vi "J1939 Editor.vi"() -> ()   [LabVIEW 2013]
doc: "This is the main VI for the configuration editor."
uses:
  Controls/StateCluster.ctl
  <vilib>/NI/Configuration Framework/Repository/NISE_CEF_Repository.lvclass
  <vilib>/NI/Configuration Framework/Node/NodeRef.ctl
  <vilib>/NI/Configuration Framework/Node/NISE_CEF_Node.lvclass
  <vilib>/NI/Configuration Framework/Node/UserEventRef.ctl
  <vilib>/NI/Configuration Framework/Controls/EventCluster.ctl
  Controls/AddMessage.ctl
  Controls/MoveMessage.ctl
  Classes/can port/can port.lvclass
  Classes/database file/database file.lvclass
  <vilib>/NI/AMC/Read Termination Message.vi
  <vilib>/NI/AMC/Create Single Message.vi
  <vilib>/NI/AMC/Update Message Routing Info.vi
  <vilib>/NI/AMC/Send Message.vi
  <vilib>/NI/AMC/Globals.vi
  <vilib>/NI/AMC/AMC.lvlib
  <vilib>/NI/Configuration Framework/NISE_CEF_TreeControl.lvlib
panel:
  in  "View":string(tree)
  in  "Exit":bool
  # "J1939 Device Configurator"
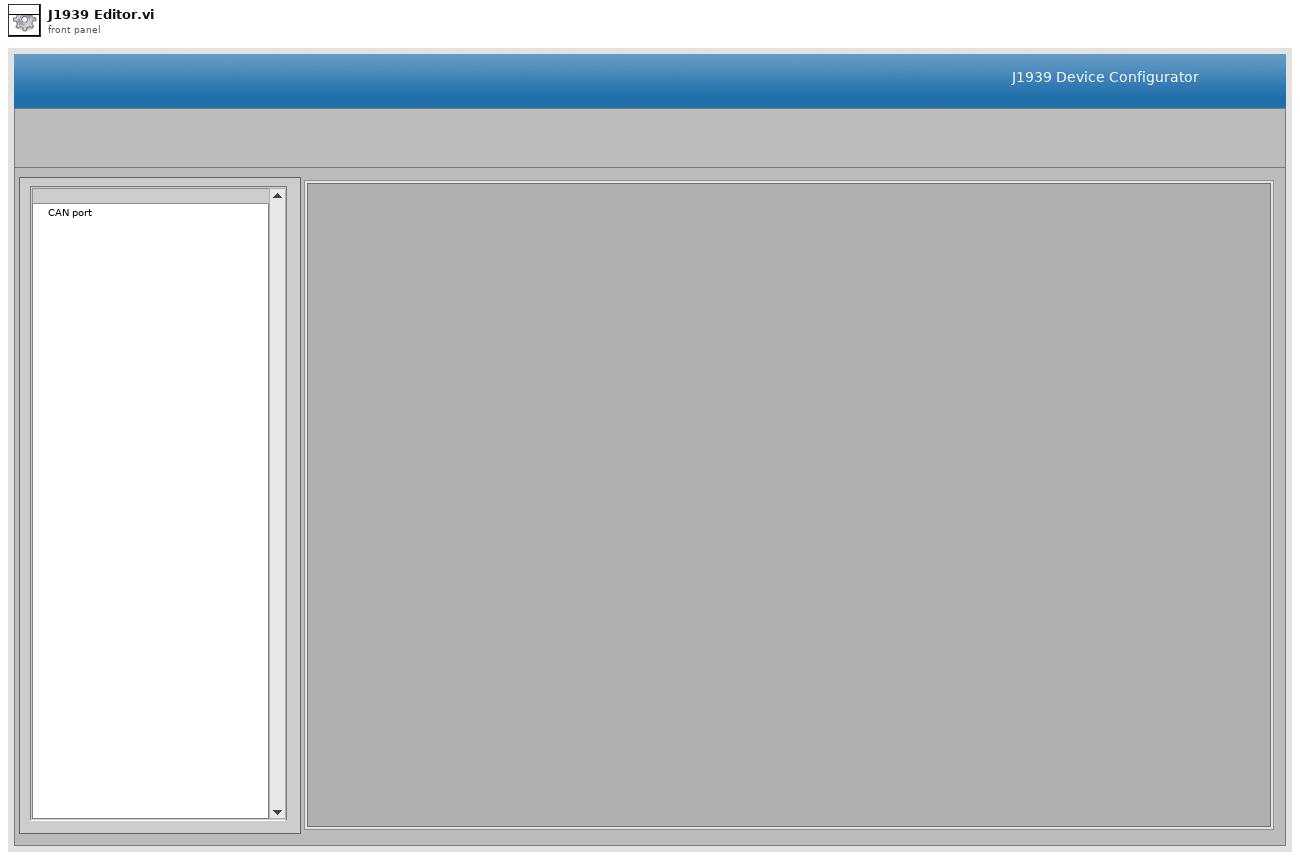
[diagram p1: front panel]
types:
  T1 = typedef "StateCluster.ctl" = cluster{"repository":refnum<class "NISE_CEF_Repository.lvclass">, "root":T2, "unsaved changes":bool, "current path":path, "user event ref":T3, "glyph path":path, "classes path":path}
  T2 = typedef "NISE_CEF_Node.lvclass/NodeRef.ctl" = refnum<data-value>
  T3 = typedef "NISE_CEF_Node.lvclass/UserEventRef.ctl" = refnum<user-event>
  T4 = typedef "AMC.lvlib/Message Queue.ctl" = refnum<queue>
  T5 = typedef "AddMessage.ctl" = cluster{"node type":string, "to add to":string}
  T6 = typedef "MoveMessage.ctl" = cluster{"node ref":T2, "new parent":T2}
  T7 = typedef "NISE_CEF_TreeControl.lvlib/EventCluster.ctl" = cluster{"command":string, "data":string}
  T8 = typedef "FilePaths.ctl" = cluster{"glyphs":path, "classes":path}
  T9 = typedef "NISE_CEF_Node.lvclass/Summary.ctl" = cluster{"ID":string, "parent ID":string, "node type":string, "text":string, "additional text":string, "glyph":string, "depth":i32, "glyph overlay":string}
  T10 = typedef "LVPoint32TypeDef.ctl" = cluster{"Horizontal":i32, "Vertical":i32}
  T11 = cluster{"data name":string, "drag data":variant}[]
  T12 = typedef "NISE_CEF_Node.lvclass/NodeMenuOptions.ctl" = cluster{"removable":bool, "movable":bool, "duplicate":bool}
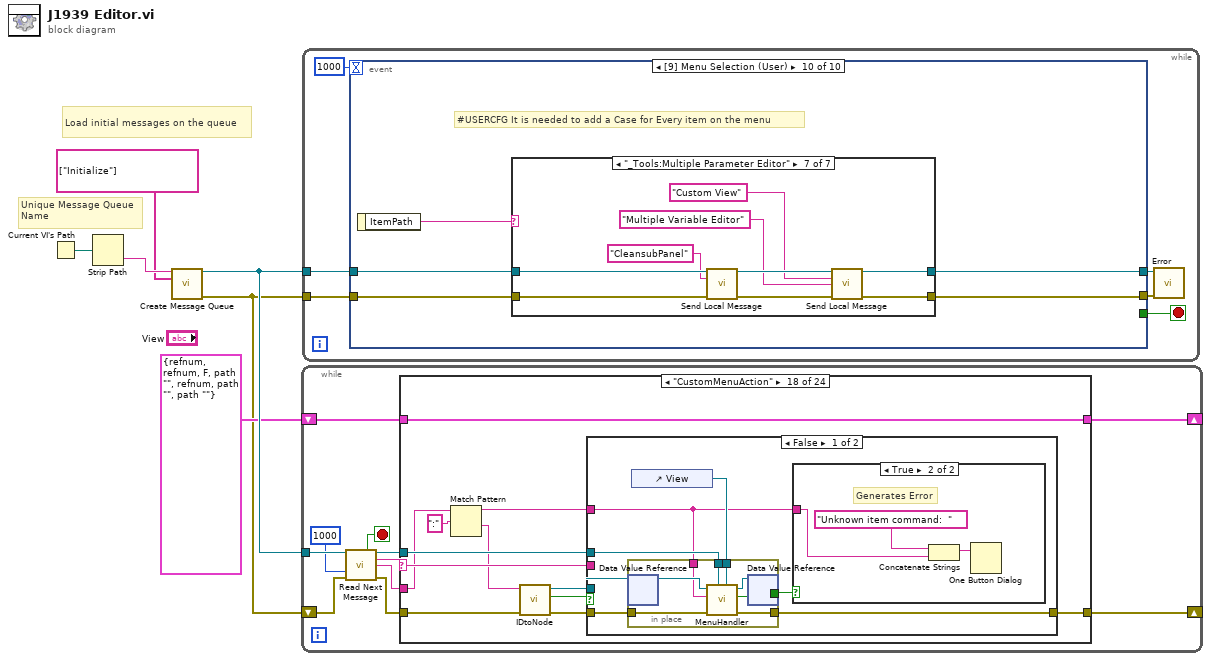
[diagram p0: block diagram]
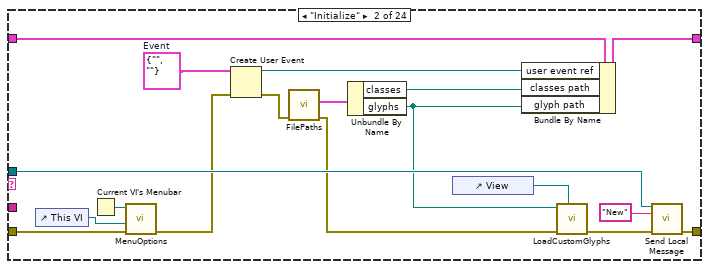
[diagram p3: hidden frame]
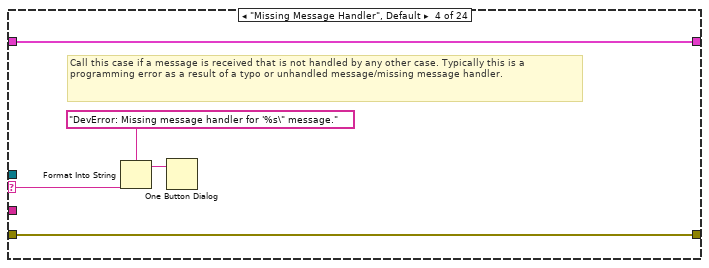
[diagram p5: hidden frame]
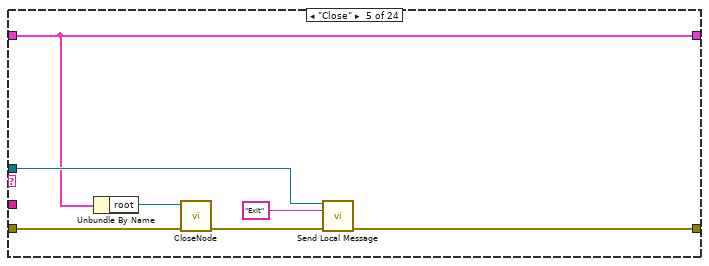
[diagram p6: hidden frame]
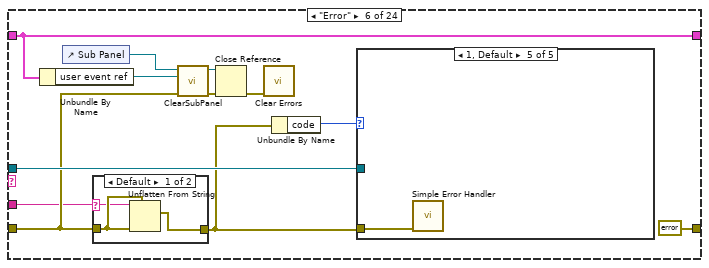
[diagram p7: hidden frame]
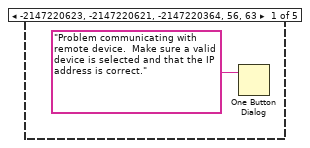
[diagram p9: hidden frame]
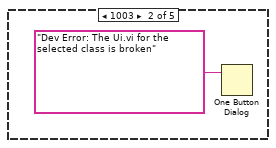
[diagram p10: hidden frame]
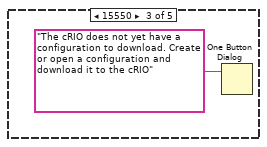
[diagram p11: hidden frame]
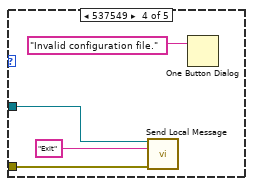
[diagram p12: hidden frame]
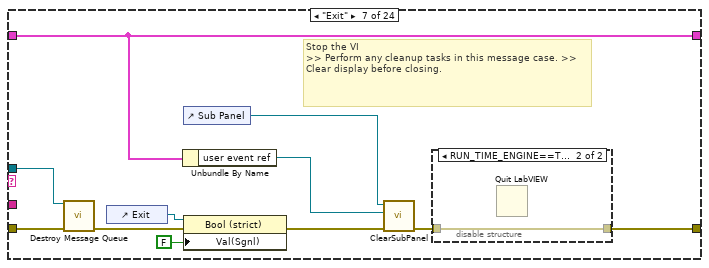
[diagram p13: hidden frame]
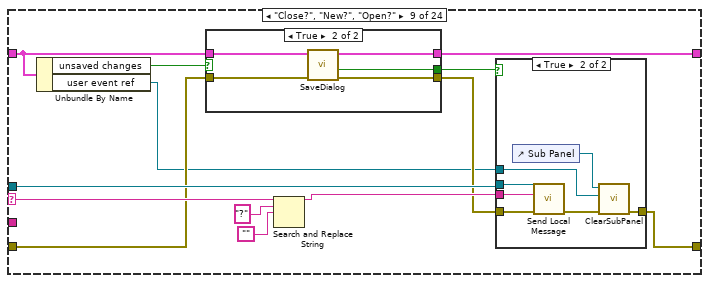
[diagram p16: hidden frame]
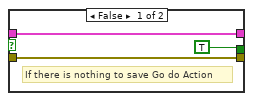
[diagram p17: hidden frame]
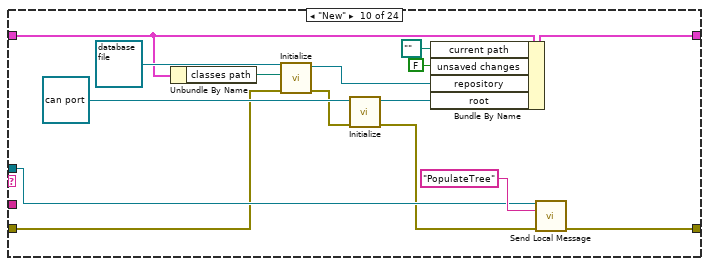
[diagram p19: hidden frame]
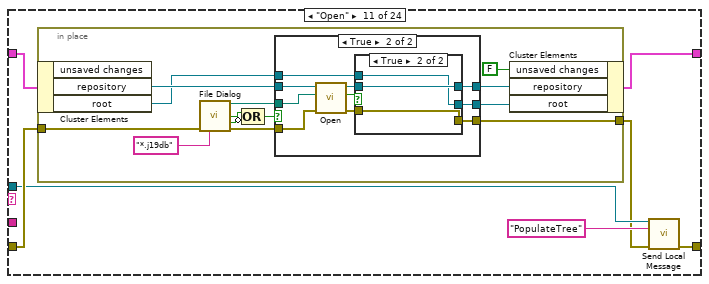
[diagram p20: hidden frame]
diagram:
  # "Unique Message Queue Name"
  # "Load initial messages on the queue"
  n1 = Current VI's Path() -> (path=w5:path)
  n2 = Strip Path(path=w5) -> (name=w6:string)  [unwired: 1 out]
  n3 = call <vilib>:"Create Message Queue.vi"("message queue name"=w6, "initial message names"=string[] ["Initialize"]) -> ("message queue out"=w3:T4, "error out"=w1:errorcluster)  [unwired: 12 in]
  n4 = while "Message Processor" {
    shift-right: [w13] -> _
    shift-left: w1 -> [w12]
    tunnel: w3 -> [w11]
    shift-right: [w9] -> _
    shift-left: T1 {"repository"=refnum, "root"=refnum, "unsaved changes"=FALSE, "current path"=path "", "user event ref"=refnum, "glyph path"=path "", "classes path"=path ""} -> [w8]
    stop <- w17 stop-if-true
    n5 = call <vilib>:"Read Next Message.vi"("message queue in"=w11, "timeout (1 ms)"=1000, "error in"=w12) -> ("exit process?"=w17:bool, "message queue out"=w7:T4, "message name"=w16:string, "message value"=w15:string, "error out"=w14:errorcluster)  [unwired: 5 in, 3 out]
    n6 = case shown="\"CustomMenuAction\"" w16 {
      selector: w16 -> [_ _ _ w41 _ _ _ _ w99 _ _ _ _ _ _ _ _ w279 _ _ _ _ _ _]
      tunnel: w15 -> [_ _ _ _ _ w52 _ _ _ _ _ _ _ w212 _ w249 w260 w277 w308 w329 _ _ w365 w385]
      tunnel: w14 -> [w19 w37 w39 w44 w46 w55 w86 w90 w92 w121 w139 w178 w204 w219 w232 w238 w259 w282 w310 w328 w345 w355 w364 w383]
      tunnel: [w19 w31 w39 w44 w50 errorcluster {"status"=FALSE, "code"=0, "source"=""} ("error out") w78 w90 w103 w133 w135 w182 w206 w216 w232 w241 w263 w285 w314 w325 w339 w350 w361 w378] -> w13
      tunnel: [w18 w26 w38 w40 w48 w60 w77 w89 w94 w131 w140 w185 w205 w213 w231 w235 w264 w286 w312 w330 w349 w354 w359 w386] -> w9
      tunnel: w8 -> [w18 w27 w38 w40 w48 w60 w77 w89 w95 w125 w141 w180 w203 w214 w231 w236 w264 w286 w313 w330 w349 w354 w359 w386]
      tunnel: w7 -> [_ w30 _ _ w49 w63 w85 _ w102 w132 w137 w181 _ w215 _ _ _ w280 _ _ _ _ w360 w377]
      frame "------------Generic Operations------------" {
        # "Dummy case to add a seperation in the Case Structure menu"
      }
      frame "Initialize" {
        w21 = T7 {"command"="", "data"=""}  # Event
        n7 = control-ref of="This VI"() -> (w36:refnum<vi>)
        n8 = Current VI's Menubar() -> (w35:refnum<k9>)
        n9 = call "MenuOptions.vi"("error in"=w37, "VI ref"=w36, "menu ref in"=w35) -> ("error out"=w25:errorcluster)  [unwired: 7 in, 1 out]
        n10 = Create User Event(user event datatype=w21, error in=w25) -> (user event=w20:refnum<user-event>, error out=w24:errorcluster)
        n11 = call "FilePaths.vi"("error in"=w24) -> ("error out"=w29:errorcluster, "paths"=w28:T8)  [unwired: 9 in]
        n12 = Unbundle By Name(w28) -> ("classes"=w23:path, "glyphs"=w22:path)
        n13 = control-ref of="View"() -> (w34:refnum<vi>)
        n14 = Bundle By Name(cluster=w27, "user event ref"=w20, "classes path"=w23, "glyph path"=w22) -> (w26:T1)
        n15 = call <vilib>:"LoadCustomGlyphs.vi"("tree ref"=w34, "error in"=w29, "glyph directory"=w22) -> ("error out"=w32:errorcluster)  [unwired: 8 in]
        n16 = call <vilib>:"Send Local Message.vi"("message queue in"=w30, "message name"="New" ("Message Name"), "error in"=w32) -> ("error out"=w31:errorcluster)  [unwired: 10 in, 2 out]
      }
      frame "", "Idle" {
      }
      frame "Missing Message Handler", Default {
        # "Call this case if a message is received that is not handled by any other case. Typically this is a programming error as a result of a typo or unhandled message/missing message handler."
        n17 = Format Into String(format string="DevError: Missing message handler for '%s\" message." ("message"), w41) -> (resulting string=w43:string)  [unwired: 2 in, 1 out]
        n18 = One Button Dialog(message=w43) -> ()  [unwired: 2 out]
      }
      frame "Close" {
        n19 = Unbundle By Name(w48) -> ("root"=w47:T2)
        n20 = call <vilib>:"CloseNode.vi"("error in"=w46, "node ref"=w47) -> ("error out"=w45:errorcluster)  [unwired: 9 in]
        n21 = call <vilib>:"Send Local Message.vi"("message queue in"=w49, "message name"="Exit", "error in"=w45) -> ("error out"=w50:errorcluster)  [unwired: 10 in, 2 out]
      }
      frame "Error" {
        n22 = Unbundle By Name(w60) -> ("user event ref"=w58:T3)
        n23 = control-ref of="Sub Panel"() -> (w59:refnum<vi>)
        n24 = case shown="Default" w52 {
          selector: w52 -> [w65 _]
          tunnel: w55 -> [w66 w67]
          tunnel: [w64 w67] -> w54
          frame Default {
            n25 = Unflatten From String(type=w66, binary string=w65, error in (no error)=w66) -> (value=w64:errorcluster)  [unwired: 2 in, 2 out]
          }
          frame "" {
          }
        }
        n26 = call <vilib>:"ClearSubPanel.vi"("error in"=w55, "user event ref"=w58, "sub panel ref in"=w59) -> ("error out"=w57:errorcluster, "sub panel ref out"=w56:refnum<vi>)  [unwired: 7 in]
        n27 = Close Reference(reference=w56, error in (no error)=w57) -> (error out=w53:errorcluster)
        n28 = call <vilib>:"Clear Errors.vi"("error in (no error)"=w53) -> ()  [unwired: 6 in, 1 out]
        n29 = Unbundle By Name(w54) -> ("code"=w61:i32)
        n30 = case shown="1, Default" w61 {
          tunnel: w63 -> [_ _ _ w73 _]
          tunnel: w54 -> [_ _ _ w72 w75]
          frame -2147220623, -2147220621, -2147220364, 56, 63 {
            n31 = One Button Dialog(message="Problem communicating with remote device.  Make sure a valid device is selected and that the IP address is correct.") -> ()  [unwired: 1 in, 1 out]
          }
          frame 1003 {
            n32 = One Button Dialog(message="Dev Error: The Ui.vi for the selected class is broken") -> ()  [unwired: 1 in, 1 out]
          }
          frame 15550 {
            n33 = One Button Dialog(message="The cRIO does not yet have a configuration to download. Create or open a configuration and download it to the cRIO") -> ()  [unwired: 1 in, 1 out]
          }
          frame 537549 {
            n34 = call <vilib>:"Send Local Message.vi"("message queue in"=w73, "message name"="Exit", "error in"=w72) -> ()  [unwired: 10 in, 3 out]
            n35 = One Button Dialog(message="Invalid configuration file.") -> ()  [unwired: 1 in, 1 out]
          }
          frame 1, Default {
            n36 = call <vilib>:"Simple Error Handler.vi"("error in (no error)"=w75) -> ()  [unwired: 1 in, 8 out]
          }
        }
      }
      frame "Exit" {
        # "Stop the VI                                                                             >> Perform any cleanup tasks in this message case. >> Clear display before closing."
        n37 = call <vilib>:"Destroy Message Queue.vi"("message queue in"=w85, "error in"=w86) -> ("error out"=w82:errorcluster)  [unwired: 11 in, 2 out]
        n38 = control-ref of="Exit"() -> (w84:refnum<vi>)
        n39 = Unbundle By Name(w77) -> ("user event ref"=w76:T3)
        n40 = control-ref of="Sub Panel"() -> (w81:refnum<vi>)
        n41 = property class="Bool (strict)"(reference=w84, error in=w82, "Val(Sgnl)"=FALSE ("Exit")) -> (error out=w80:errorcluster)  [unwired: 1 out]
        n42 = call <vilib>:"ClearSubPanel.vi"("error in"=w80, "user event ref"=w76, "sub panel ref in"=w81) -> ("error out"=w79:errorcluster)  [unwired: 7 in, 1 out]
        n43 = disable-structure shown="RUN_TIME_ENGINE==True" {
          disable-tunnel: [w87 w88] -> w78
          disable-tunnel: w79 -> [w87 w88]
          frame condition #0 (active) {
          }
          frame condition #1 {
            n44 = Quit LabVIEW() -> ()  [unwired: 1 in]
          }
        }
      }
      frame "------------Menu Operations--------------" {
        # "Dummy case to add a seperation in the Case Structure menu"
      }
      frame "Close?", "New?", "Open?" {
        n45 = Unbundle By Name(w95) -> ("unsaved changes"=w97:bool, "user event ref"=w91:T3)
        n46 = case shown="True" w97 {
          tunnel: [TRUE ("SaveFlag") w111] -> w96
          tunnel: w95 -> [w105 w110]
          tunnel: [w105 w109] -> w94
          tunnel: w92 -> [w104 w108]
          tunnel: [w104 w107] -> w93
          frame False {
            # "If there is nothing to save Go do Action"
          }
          frame True {
            n47 = call "SaveDialog.vi"("error in"=w108, "state in"=w110) -> ("error out"=w107:errorcluster, "new"=w111:bool, "state out"=w109:T1)  [unwired: 7 in]
          }
        }
        n48 = Search and Replace String(input string=w99, search string="?", replace string="") -> (result string=w98:string)  [unwired: 5 in, 3 out]
        n49 = case shown="True" w96 {
          tunnel: w93 -> [w112 w119]
          tunnel: [w112 w115] -> w103
          tunnel: w102 -> [_ w118]
          tunnel: w98 -> [_ w117]
          tunnel: w91 -> [_ w114]
          frame False {
          }
          frame True {
            n50 = control-ref of="Sub Panel"() -> (w113:refnum<vi>)
            n51 = call <vilib>:"Send Local Message.vi"("message queue in"=w118, "message name"=w117, "error in"=w119) -> ("error out"=w116:errorcluster)  [unwired: 10 in, 2 out]
            n52 = call <vilib>:"ClearSubPanel.vi"("error in"=w116, "user event ref"=w114, "sub panel ref in"=w113) -> ("error out"=w115:errorcluster)  [unwired: 7 in, 1 out]
          }
        }
      }
      frame "New" {
        n53 = Unbundle By Name(w125) -> ("classes path"=w124:path)
        n54 = call-dynamic "Initialize.vi"("error in"=w121, "path"=w124, "repository in"=refnum<class "database file.lvclass"> refnum ("cRIORepo.lvclass")) -> ("error out"=w123:errorcluster, "repository out"=w126:refnum<class "database file.lvclass">)  [unwired: 7 in]
        n55 = call-dynamic "Initialize.vi"("error in"=w123, "cRIO in"=refnum<class "can port.lvclass"> refnum ("cRIO.lvclass")) -> ("error out"=w122:errorcluster, "data value reference"=w128:T2)  [unwired: 7 in, 1 out]
        n56 = Bundle By Name(cluster=w125, "current path"=path "", "unsaved changes"=FALSE ("SaveFlag"), "repository"=w126, "root"=w128) -> (w131:T1)
        n57 = call <vilib>:"Send Local Message.vi"("message queue in"=w132, "message name"="PopulateTree", "error in"=w122) -> ("error out"=w133:errorcluster)  [unwired: 10 in, 2 out]
      }
      frame "Open" {
        n58 = in-place {
          in-place-border: w139 -> [w147]
          in-place-border: [w151] -> w136
          n59 = in-place-cluster #1(w141) -> ("repository"=w154:refnum<class "NISE_CEF_Repository.lvclass">, "root"=w145:T2)  [unwired: 1 out]
          n60 = call "File Dialog"("error in"=w147, "pattern (all files)"="*.j19db") -> ("selected path"=w148:path, "exists"=w144:bool, "cancelled"=w143:bool, "error out"=w146:errorcluster)  [unwired: 10 in]
          n61 = Compound Arithmetic op=OR(w144, invert w143) -> (w142:bool)
          n62 = case shown="True" w142 {
            tunnel: w154 -> [w155 w167]
            tunnel: [w155 w165] -> w152
            tunnel: [w156 w163] -> w151
            tunnel: [w157 w162] -> w150
            tunnel: w148 -> [_ w160]
            tunnel: w146 -> [w156 w159]
            tunnel: w145 -> [w157 w158]
            frame False {
            }
            frame True {
              n63 = call-dynamic "Open.vi"("error in"=w159, "file path"=w160, "repository in"=w167) -> ("error out"=w164:errorcluster, "invalid?"=w161:bool, "repository out"=w166:refnum<class "NISE_CEF_Repository.lvclass">)  [unwired: 6 in]
              n64 = case shown="True" w161 {
                tunnel: w166 -> [w172 w175]
                tunnel: [w171 w175] -> w165
                tunnel: w164 -> [w170 w174]
                tunnel: [w169 w174] -> w163
                tunnel: [w168 w173] -> w162
                tunnel: w158 -> [_ w173]
                frame False {
                  n65 = call-dynamic "WriteTree.vi"("error in"=w170, "repository in"=w172) -> ("error out"=w169:errorcluster, "root"=w168:T2, "repository out"=w171:refnum<class "NISE_CEF_Repository.lvclass">)  [unwired: 7 in]
                }
                frame True {
                }
              }
            }
          }
          n66 = in-place-cluster #1("unsaved changes"=FALSE ("SaveFlag"), "repository"=w152, "root"=w150) -> (w140:T1)
        }
        n67 = call <vilib>:"Send Local Message.vi"("message queue in"=w137, "message name"="PopulateTree", "error in"=w136) -> ("error out"=w135:errorcluster)  [unwired: 10 in, 2 out]
      }
      frame "Save" {
        n68 = in-place {
          in-place-border: w178 -> [w189]
          in-place-border: [w188] -> w177
          in-place-border: [w186] -> w176
          n69 = in-place-cluster #2(w180) -> ("current path"=w187:path, "root"=w190:T2, "repository"=w192:refnum<class "NISE_CEF_Repository.lvclass">)
          n70 = Empty String/Path?(string/path=w187) -> (empty?=w186:bool)
          n71 = call-dynamic "ReadTree.vi"("error in"=w189, "root"=w190, "repository in"=w192) -> ("error out"=w188:errorcluster, "repository out"=w191:refnum<class "NISE_CEF_Repository.lvclass">)  [unwired: 7 in]
          n72 = in-place-cluster #2("current path"=w187, "root"=w190, "repository"=w191) -> (w179:T1)
        }
        n73 = case shown="True" w176 {
          tunnel: w179 -> [w196 w198]
          tunnel: [w195 w197] -> w185
          tunnel: [w194 w199] -> w183
          tunnel: w177 -> [w193 w200]
          frame False {
            n74 = call "Save.vi"("error in"=w193, "state in"=w196) -> ("error out"=w194:errorcluster, "state out"=w195:T1)  [unwired: 8 in]
          }
          frame True {
            # "Empty path use Dialog"
            n75 = call "SaveAs.vi"("error in"=w200, "state in"=w198) -> ("error out"=w199:errorcluster, "state out"=w197:T1)  [unwired: 7 in, 1 out]
          }
        }
        n76 = call <vilib>:"Send Local Message.vi"("message queue in"=w181, "message name"="PopulateTree", "error in"=w183) -> ("error out"=w182:errorcluster)  [unwired: 10 in, 2 out]
      }
      frame "SaveAs" {
        n77 = in-place {
          in-place-border: w204 -> [w208]
          in-place-border: [w207] -> w202
          n78 = in-place-cluster #3(w203) -> ("root"=w209:T2, "repository"=w211:refnum<class "NISE_CEF_Repository.lvclass">)
          n79 = call-dynamic "ReadTree.vi"("error in"=w208, "root"=w209, "repository in"=w211) -> ("error out"=w207:errorcluster, "repository out"=w210:refnum<class "NISE_CEF_Repository.lvclass">)  [unwired: 7 in]
          n80 = in-place-cluster #3("root"=w209, "repository"=w210) -> (w201:T1)
        }
        n81 = call "SaveAs.vi"("error in"=w202, "state in"=w201) -> ("error out"=w206:errorcluster, "state out"=w205:T1)  [unwired: 7 in, 1 out]
      }
      frame "Custom View" {
        n82 = in-place {
          in-place-border: w219 -> [w230]
          in-place-border: [w229] -> w217
          in-place-border: w212 -> [w220]
          n83 = in-place-cluster #4(w214) -> ("repository"=w224:refnum<class "NISE_CEF_Repository.lvclass">, "root"=w223:T2)
          n84 = call-dynamic "ReadTree.vi"("error in"=w230, "root"=w223, "repository in"=w224) -> ("error out"=w227:errorcluster, "repository out"=w226:refnum<class "NISE_CEF_Repository.lvclass">)  [unwired: 7 in]
          n85 = call-dynamic "CustomView.vi"("error in"=w227, "view name"=w220, "repository in"=w226) -> ("error out"=w228:errorcluster, "repository out"=w225:refnum<class "NISE_CEF_Repository.lvclass">)  [unwired: 7 in]
          n86 = call-dynamic "WriteTree.vi"("error in"=w228, "repository in"=w225) -> ("error out"=w229:errorcluster, "root"=w221:T2, "repository out"=w222:refnum<class "NISE_CEF_Repository.lvclass">)  [unwired: 7 in]
          n87 = in-place-cluster #4("repository"=w222, "root"=w221) -> (w213:T1)
        }
        n88 = call <vilib>:"Send Local Message.vi"("message queue in"=w215, "message name"="PopulateTree", "error in"=w217) -> ("error out"=w216:errorcluster)  [unwired: 10 in, 2 out]
      }
      frame "-------TreeControl Operations-----------" {
        # "Dummy case to add a seperation in the Case Structure menu"
      }
      frame "AddNode" {
        n89 = Unflatten From String(type=T5 {"node type"="", "to add to"=""} ("input cluster"), binary string=w249) -> (value=w247:T5)  [unwired: 3 in, 2 out]
        n90 = Unbundle By Name(w247) -> ("to add to"=w244:string, "node type"=w234:string)
        n91 = in-place {
          in-place-border: w238 -> [w255]
          in-place-border: [w254] -> w237
          in-place-border: w234 -> [w253]
          in-place-border: [w252] -> w233
          n92 = in-place-cluster #5(w236) -> ("repository"=w257:refnum<class "NISE_CEF_Repository.lvclass">)
          n93 = call-dynamic "GetClassPath.vi"("error in"=w255, "class name"=w253, "Repository in"=w257) -> ("error out"=w254:errorcluster, "class path"=w252:path, "Repository out"=w256:refnum<class "NISE_CEF_Repository.lvclass">)  [unwired: 6 in]
          n94 = in-place-cluster #5("repository"=w256) -> (w235:T1)
        }
        n95 = control-ref of="View"() -> (w239:refnum<vi>)
        n96 = call <vilib>:"Get LV Class Default Value.vi"("error in (no error)"=w237, "class path"=w233) -> ("error out"=w250:errorcluster, "object"=w251:refnum<class>)  [unwired: 8 in]
        n97 = To More Specific Class(target class=refnum<class "NISE_CEF_Node.lvclass"> refnum ("Node.lvclass"), reference=w251, error in=w250) -> (specific class reference=w246:refnum<class "NISE_CEF_Node.lvclass">, error out=w243:errorcluster)
        n98 = call <vilib>:"AddNode.vi"("error in"=w243, "node in"=w246, "parent node ID"=w244) -> ("error out"=w242:errorcluster, "summary"=w240:T9[])  [unwired: 7 in]
        n99 = call <vilib>:"PopulateTreeSumary.vi"("error in"=w242, "array"=w240, "tree ref in"=w239) -> ("error out"=w241:errorcluster)  [unwired: 8 in]
      }
      frame "Duplicate" {
        n100 = call <vilib>:"IDtoNode.vi"("error in"=w259, "ID"=w260) -> ("error out"=w261:errorcluster, "invalid Id"=w258:bool, "node ref"=w262:T2)  [unwired: 7 in]
        n101 = case shown="False" w258 {
          tunnel: [w273 w274] -> w263
          tunnel: w262 -> [w271 _]
          tunnel: w261 -> [w268 w274]
          frame False {
            n102 = call <vilib>:"DuplicateNode.vi"("same parent?"=TRUE ("s"), "error in"=w268, "node ref in"=w271) -> ("error out"=w269:errorcluster, "new node ref"=w270:T2)  [unwired: 7 in]
            n103 = call <vilib>:"Summary.vi"("error in"=w269, "node self ref"=w270) -> ("error out"=w266:errorcluster, "summary"=w265:T9[])  [unwired: 8 in]
            n104 = control-ref of="View"() -> (w272:refnum<vi>)
            n105 = call <vilib>:"PopulateTreeSumary.vi"("error in"=w266, "array"=w265, "tree ref in"=w272) -> ("error out"=w273:errorcluster)  [unwired: 8 in]
          }
          frame True {
          }
        }
      }
      frame "CustomMenuAction" {
        n106 = Match Pattern(string=w277, regular expression=":") -> (before substring=w276:string, after substring=w275:string)  [unwired: 1 in, 2 out]
        n107 = call <vilib>:"IDtoNode.vi"("error in"=w282, "ID"=w275) -> ("error out"=w283:errorcluster, "invalid Id"=w281:bool, "node ref"=w284:T2)  [unwired: 7 in]
        n108 = case shown="False" w281 {
          tunnel: [w290 w305] -> w285
          tunnel: w284 -> [w287 _]
          tunnel: w283 -> [w291 w305]
          tunnel: w280 -> [w293 _]
          tunnel: w279 -> [_ _]
          tunnel: w276 -> [w288 _]
          frame False {
            n109 = control-ref of="View"() -> (w292:refnum<vi>)
            n110 = in-place {
              in-place-border: w293 -> [w303]
              in-place-border: w292 -> [w301]
              in-place-border: w291 -> [w300]
              in-place-border: [w299] -> w290
              in-place-border: [w298] -> w289
              in-place-border: w288 -> [w297]
              n111 = in-place-dvr #6(w287) -> (w304:refnum<class "NISE_CEF_Node.lvclass">)  [unwired: 1 out]
              n112 = call-dynamic "MenuHandler.vi"("tree control"=w301, "main message queue"=w303, "error in"=w300, "menu string"=w297, "NISE_CEF_Node in"=w304) -> ("error out"=w299:errorcluster, "Unhandled"=w298:bool, "NISE_CEF_Node out"=w302:refnum<class "NISE_CEF_Node.lvclass">)  [unwired: 3 in, 1 out]
              n113 = in-place-dvr #6(w302) -> ()  [unwired: 2 out]
            }
            n114 = case shown="True" w289 {
              tunnel: w288 -> [_ w294]
              frame False {
              }
              frame True {
                # "Generates Error"
                n115 = Concatenate Strings("Unknown item command:  " ("message"), w294) -> (w296:string)
                n116 = One Button Dialog(message=w296) -> ()  [unwired: 1 in, 1 out]
              }
            }
          }
          frame True {
          }
        }
      }
      frame "RefreshNode" {
        # "Refreshes the node in the Tree               Sets the save flag to true                       This case can be called from the UIs of the nodes"
        n117 = call <vilib>:"IDtoNode.vi"("error in"=w310, "ID"=w308) -> ("error out"=w309:errorcluster, "invalid Id"=w306:bool, "node ref"=w307:T2)  [unwired: 7 in]
        n118 = case shown="True" w306 {
          tunnel: [w321 w323] -> w314
          tunnel: w309 -> [w316 w323]
          tunnel: w307 -> [w315 _]
          frame False {
            n119 = call <vilib>:"Summary.vi"("error in"=w316, "node self ref"=w315) -> ("error out"=w318:errorcluster, "summary"=w317:T9[])  [unwired: 8 in]
            n120 = control-ref of="View"() -> (w319:refnum<vi>)
            n121 = call <vilib>:"RefreshSubTree.vi"("error in"=w318, "node information"=w317, "tree ref in"=w319) -> ("error out"=w322:errorcluster, "tree ref out"=w320:refnum<vi>)  [unwired: 7 in]
            n122 = Close Reference(reference=w320, error in (no error)=w322) -> (error out=w321:errorcluster)
          }
          frame True {
          }
        }
        n123 = Bundle By Name(cluster=w313, "unsaved changes"=TRUE ("SaveFlag")) -> (w312:T1)
      }
      frame "RemoveNode" {
        n124 = call <vilib>:"IDtoNode.vi"("error in"=w328, "ID"=w329) -> ("error out"=w327:errorcluster, "invalid Id"=w324:bool, "node ref"=w326:T2)  [unwired: 7 in]
        n125 = case shown="False" w324 {
          tunnel: w327 -> [w336 w337]
          tunnel: w326 -> [w335 _]
          tunnel: [w331 w337] -> w325
          frame False {
            n126 = call <vilib>:"RemoveNode.vi"("error in"=w336, "node"=w335) -> ("error out"=w332:errorcluster, "node ID"=w334:string)  [unwired: 8 in]
            n127 = control-ref of="View"() -> (w333:refnum<vi>)
            n128 = call <vilib>:"ClearTreeNode.vi"("error in"=w332, "tag"=w334, "tree reference"=w333) -> ("error out"=w331:errorcluster)  [unwired: 8 in]
          }
          frame True {
          }
        }
      }
      frame "PopulateTree" {
        n129 = Unbundle By Name(w349) -> ("user event ref"=w338:T3, "root"=w343:T2)
        n130 = call <vilib>:"Summary.vi"("error in"=w345, "depth"=0 ("Depth"), "node self ref"=w343) -> ("error out"=w344:errorcluster, "summary"=w348:T9[])  [unwired: 7 in]
        n131 = control-ref of="This VI"() -> (w346:refnum<vi>)
        n132 = control-ref of="View"() -> (w347:refnum<vi>)
        n133 = call <vilib>:"RefreshEntireTree.vi"("calling VI in"=w346, "error in"=w344, "array"=w348, "tree ref in"=w347) -> ("error out"=w340:errorcluster)  [unwired: 7 in]
        n134 = control-ref of="Sub Panel"() -> (w341:refnum<vi>)
        n135 = call <vilib>:"ClearSubPanel.vi"("error in"=w340, "user event ref"=w338, "sub panel ref in"=w341) -> ("error out"=w339:errorcluster)  [unwired: 7 in, 1 out]
      }
      frame "CleansubPanel" {
        n136 = Unbundle By Name(w354) -> ("user event ref"=w353:T3)
        n137 = control-ref of="Sub Panel"() -> (w356:refnum<vi>)
        n138 = call <vilib>:"ClearSubPanel.vi"("error in"=w355, "user event ref"=w353, "sub panel ref in"=w356) -> ("error out"=w352:errorcluster, "sub panel ref out"=w351:refnum<vi>)  [unwired: 7 in]
        n139 = Close Reference(reference=w351, error in (no error)=w352) -> (error out=w350:errorcluster)
      }
      frame "ActivateNode" {
        n140 = Unbundle By Name(w359) -> ("user event ref"=w358:T3)
        n141 = call <vilib>:"IDtoNode.vi"("error in"=w364, "ID"=w365) -> ("error out"=w357:errorcluster, "invalid Id"=w363:bool, "node ref"=w362:T2)  [unwired: 7 in]
        n142 = case shown="False" w363 {
          tunnel: w362 -> [w372 _]
          tunnel: [w373 w374] -> w361
          tunnel: w357 -> [w370 w374]
          tunnel: w360 -> [w367 _]
          tunnel: w358 -> [w368 _]
          frame False {
            n143 = control-ref of="Sub Panel"() -> (w369:refnum<vi>)
            n144 = call <vilib>:"ClearSubPanel.vi"("error in"=w370, "user event ref"=w368, "sub panel ref in"=w369) -> ("error out"=w371:errorcluster, "sub panel ref out"=w366:refnum<vi>)  [unwired: 7 in]
            n145 = call <vilib>:"LoadNodeUI.vi"("user event out"=w368, "error in"=w371, "sub panel ref in"=w366, "main queue"=w367, "node"=w372) -> ("error out"=w373:errorcluster)  [unwired: 6 in]
          }
          frame True {
          }
        }
      }
      frame "Move" {
        n146 = Unflatten From String(type=T6 {"node ref"=refnum, "new parent"=refnum} ("Cluster"), binary string=w385, error in (no error)=w383) -> (value=w382:T6, error out=w381:errorcluster)  [unwired: 2 in, 1 out]
        n147 = Unbundle By Name(w382) -> ("node ref"=w376:T2, "new parent"=w375:T2)
        n148 = call <vilib>:"MoveNode.vi"("error in"=w381, "new parent"=w375, "node"=w376) -> ("error out"=w379:errorcluster)  [unwired: 8 in]
        n149 = call <vilib>:"Send Local Message.vi"("message queue in"=w377, "message name"="PopulateTree", "error in"=w379) -> ("error out"=w378:errorcluster)  [unwired: 10 in, 2 out]
      }
    }
  }
  n150 = while "User Interface Event Handler" {
    tunnel: w3 -> [w391]
    tunnel: w1 -> [w387]
    stop <- w390 stop-if-true
    n151 = event shown="[9] Menu Selection (User)" {
      selector: _ -> [_ _ _ _ _ _ _ _ _ _]
      dyn-events: _ -> [_ _ _ _ _ _ _ _ _ _]
      timeout: 1000 -> [_ _ _ _ _ _ _ _ _ _]
      tunnel: w391 -> [w394 w402 w426 w478 w506 w513 w542 w546 w556 w561]
      tunnel: [_ _ _ _ TRUE _ _ _ _ _] -> w390
      tunnel: [w394 w402 w423 w476 w502 w513 w539 w546 w554 w560] -> w389
      tunnel: [w393 w398 w422 w475 w503 w509 w538 w543 w552 w558] -> w388
      tunnel: w387 -> [w393 w401 w421 w477 w504 w512 w537 w545 w553 w559]
      event Timeout {
        # "Timeout code can be added here for autosave or Lock Screen"
        n152 = event-data() -> ()  [unwired: 1 in, 1 out]
      }
      event "View": Shortcut Menu Activation? {
        n153 = event-data() -> ("CtlRef"=w408:refnum<vi>, "Coords"=w407:T10, "MenuRef"=w404:refnum<k9>)  [unwired: 1 in]
        n154 = invoke class="Tree (strict)" method="Point To Row Column"(reference=w408, error in=w401, "Point"=w407) -> (error out=w400:errorcluster, "Tag"=w406:string)  [unwired: 5 in, 6 out]
        n155 = call <vilib>:"IDtoNode.vi"("error in"=w400, "ID"=w406) -> ("error out"=w396:errorcluster, "invalid Id"=w403:bool, "node ref"=w405:T2)  [unwired: 7 in]
        n156 = case shown="False" w403 {
          tunnel: w405 -> [w413 _]
          tunnel: w404 -> [w412 _]
          tunnel: [w411 _] -> w399
          tunnel: [w410 _] -> w397
          tunnel: w396 -> [w409 w419]
          tunnel: [w409 w419] -> w395
          frame False {
            n157 = in-place {
              in-place-border: w412 -> [w416]
              in-place-border: [w414] -> w411
              n158 = in-place-dvr #7(w413) -> (w418:refnum<class "NISE_CEF_Node.lvclass">, w415:errorcluster)
              n159 = call-dynamic "ShortcutMenu.vi"("error in"=w415, "menu ref in"=w416, "node in"=w418) -> ("error out"=w414:errorcluster, "node out"=w417:refnum<class "NISE_CEF_Node.lvclass">)  [unwired: 6 in, 1 out]
              n160 = in-place-dvr #7(w417) -> (w410:errorcluster)  [unwired: 1 out]
            }
          }
          frame True {
          }
        }
        n161 = Merge Errors(w397, w399, w395) -> (w398:errorcluster)
        n162 = event-data() -> ()  [unwired: 2 in, 1 out]
      }
      event "View": Shortcut Menu Selection (User) {
        n163 = event-data() -> ("ItemPath"=w425:string, "CtlRef"=w429:refnum<vi>, "Coords"=w430:T10)  [unwired: 1 in]
        n164 = invoke class="Tree (strict)" method="Point To Row Column"(reference=w429, error in=w421, "Point"=w430) -> (error out=w420:errorcluster, "Tag"=w424:string)  [unwired: 5 in, 6 out]
        n165 = Match Pattern(string=w425, regular expression=":") -> (before substring=w428:string, after substring=w427:string)  [unwired: 1 in, 2 out]
        n166 = case shown="Default" w428 {
          selector: w428 -> [w432 _ _ _]
          tunnel: w427 -> [_ _ _ w457]
          tunnel: w426 -> [w439 w446 w452 w459]
          tunnel: w424 -> [w434 w444 w450 w458]
          tunnel: [w436 w443 w449 w455] -> w423
          tunnel: [w437 w442 w447 w453] -> w422
          tunnel: w420 -> [w438 w441 w448 w454]
          frame Default {
            n167 = Concatenate Strings(w432, ":" ("string"), w434) -> (w435:string)
            n168 = call <vilib>:"Send Local Message.vi"("message queue in"=w439, "message name"="CustomMenuAction" ("Message Name"), "message value"=w435, "error in"=w438) -> ("message queue out"=w436:T4, "error out"=w437:errorcluster)  [unwired: 9 in, 1 out]
          }
          frame "Remove" {
            n169 = call <vilib>:"Send Local Message.vi"("message queue in"=w446, "message name"="RemoveNode" ("Message Name"), "message value"=w444, "error in"=w441) -> ("message queue out"=w443:T4, "error out"=w442:errorcluster)  [unwired: 9 in, 1 out]
          }
          frame "Duplicate" {
            n170 = call <vilib>:"Send Local Message.vi"("message queue in"=w452, "message name"="Duplicate" ("Message Name"), "message value"=w450, "error in"=w448) -> ("message queue out"=w449:T4, "error out"=w447:errorcluster)  [unwired: 9 in, 1 out]
          }
          frame "Add" {
            n171 = Bundle By Name(cluster=T5 {"node type"="", "to add to"=""} ("input cluster"), "node type"=w457, "to add to"=w458) -> (w460:T5)
            n172 = Flatten To String(anything=w460) -> (data string=w461:string)  [unwired: 3 in, 2 out]
            n173 = call <vilib>:"Send Local Message.vi"("message queue in"=w459, "message name"="AddNode" ("Message Name"), "message value"=w461, "error in"=w454) -> ("message queue out"=w455:T4, "error out"=w453:errorcluster)  [unwired: 9 in, 1 out]
          }
        }
      }
      event "View": Drop {
        n174 = event-data() -> ("CtlRef"=w481:refnum<vi>, "Coords"=w480:T10)  [unwired: 1 in]
        n175 = invoke class="Tree (strict)" method="Point To Row Column"(reference=w481, error in=w477, "Point"=w480) -> (reference out=w479:refnum<vi>, error out=w474:errorcluster, "Tag"=w471:string)  [unwired: 5 in, 5 out]
        n176 = call <vilib>:"ValidDragDrop.vi"("error in"=w474, "drag over"=w471, "Tree Ref in"=w479) -> ("Error Out"=w466:errorcluster, "Accepted"=w469:bool, "Drag"=w473:string, "Tree Ref out"=w483:refnum<vi>)  [unwired: 1 in, 4 out]
        n177 = call <vilib>:"IDtoNode.vi"("error in"=w466, "ID"=w471) -> ("error out"=w467:errorcluster, "invalid Id"=w464:bool, "node ref"=w470:T2)  [unwired: 7 in]
        n178 = call <vilib>:"IDtoNode.vi"("error in"=w467, "ID"=w473) -> ("error out"=w465:errorcluster, "invalid Id"=w463:bool, "node ref"=w472:T2)  [unwired: 7 in]
        n179 = Compound Arithmetic op=AND(w469, invert w464, invert w463) -> (w468:bool)
        n180 = case shown="True" w468 {
          tunnel: w473 -> [_ w499]
          tunnel: w483 -> [_ w501]
          tunnel: [_ TRUE] -> w482
          tunnel: w471 -> [_ w497]
          tunnel: w478 -> [w485 w496]
          tunnel: [w485 w492] -> w476
          tunnel: [w484 w491] -> w475
          tunnel: w472 -> [_ w487]
          tunnel: w470 -> [_ w486]
          tunnel: w465 -> [w484 w488]
          frame False {
          }
          frame True {
            n181 = invoke class="Tree (strict)" method="Edit Tree Items.Move Item"(reference=w501, error in=w488, "tag"=w499, "New Parent"=w497) -> (error out=w489:errorcluster)  [unwired: 3 in, 6 out]
            n182 = Bundle By Name(cluster=T6 {"node ref"=refnum, "new parent"=refnum} ("Cluster"), "new parent"=w486, "node ref"=w487) -> (w495:T6)
            n183 = Flatten To String(anything=w495, error in (no error)=w489) -> (data string=w494:string, error out=w490:errorcluster)  [unwired: 2 in, 1 out]
            n184 = call <vilib>:"Send Local Message.vi"("message queue in"=w496, "message name"="Move", "message value"=w494, "error in"=w490) -> ("message queue out"=w492:T4, "error out"=w491:errorcluster)  [unwired: 9 in, 1 out]
          }
        }
        n185 = event-data("Accepted?"=w482) -> ()  [unwired: 1 in, 1 out]
      }
      event "Exit": Value Change {
        # "Exit the application                                           >> Stop this message generator loop    Cleaning errors if the other loop stop this one"
        n186 = event-data() -> ()  [unwired: 1 in, 1 out]
        n187 = call <vilib>:"Send Local Message.vi"("message queue in"=w506, "message name"="Close", "error in"=w504) -> ("message queue out"=w502:T4, "error out"=w507:errorcluster)  [unwired: 10 in, 1 out]
        n188 = call <vilib>:"Clear Errors.vi"("error in (no error)"=w507) -> ("error out"=w503:errorcluster)  [unwired: 6 in]
      }
      event "View": Drag Starting? {
        n189 = event-data() -> ("Data"=w519:T11, "CtlRef"=w521:refnum<vi>, "Coords"=w520:T10)  [unwired: 1 in]
        n190 = invoke class="Tree (strict)" method="Point To Row Column"(reference=w521, error in=w512, "Point"=w520) -> (error out=w511:errorcluster, "Tag"=w518:string)  [unwired: 5 in, 6 out]
        n191 = call <vilib>:"IDtoNode.vi"("error in"=w511, "ID"=w518) -> ("error out"=w510:errorcluster, "invalid Id"=w517:bool, "node ref"=w516:T2)  [unwired: 7 in]
        n192 = case shown="False" w517 {
          tunnel: w516 -> [w529 _]
          tunnel: [w526 TRUE ("Removable")] -> w514
          tunnel: w510 -> [w525 w535]
          tunnel: [w522 w535] -> w509
          frame False {
            n193 = in-place {
              in-place-border: [w532] -> w528
              in-place-border: w525 -> [w531]
              in-place-border: [w530] -> w524
              n194 = in-place-dvr #8(w529) -> (w534:refnum<class "NISE_CEF_Node.lvclass">)  [unwired: 1 out]
              n195 = call-dynamic "EditOptions.vi"("error in"=w531, "node in"=w534) -> ("error out"=w530:errorcluster, "edit options"=w532:T12, "node out"=w533:refnum<class "NISE_CEF_Node.lvclass">)  [unwired: 6 in, 1 out]
              n196 = in-place-dvr #8(w533) -> (w523:errorcluster)  [unwired: 1 out]
            }
            n197 = Unbundle By Name(w528) -> ("movable"=w527:bool)
            n198 = Merge Errors(w523, w524) -> (w522:errorcluster)
            n199 = Not(x=w527) -> (.not. x?=w526:bool)
          }
          frame True {
          }
        }
        n200 = event-data("Data"=w519, "Drag Mode"=enum32{"copy or move", "copy only", "move only"}."move only", "Discard?"=w514) -> ()  [unwired: 1 in, 1 out]
      }
      event "View": Value Change {
        n201 = event-data() -> ("NewVal"=w540:string)  [unwired: 1 in]
        n202 = call <vilib>:"Send Local Message.vi"("message queue in"=w542, "message name"="ActivateNode" ("Message Name"), "message value"=w540, "error in"=w537) -> ("message queue out"=w539:T4, "error out"=w538:errorcluster)  [unwired: 9 in, 1 out]
      }
      event "View": event type 3.0.xa000003a {
        n203 = event-data() -> ("CtlRef"=w551:refnum<vi>, "Coords"=w548:T10)  [unwired: 1 in]
        n204 = invoke class="Tree (strict)" method="Point To Row Column"(reference=w551, error in=w545, "Point"=w548) -> (reference out=w550:refnum<vi>, error out=w544:errorcluster, "Tag"=w549:string)  [unwired: 5 in, 5 out]
        n205 = call <vilib>:"ValidDragDrop.vi"("error in"=w544, "drag over"=w549, "Tree Ref in"=w550) -> ("Error Out"=w543:errorcluster, "Accepted"=w547:bool)  [unwired: 1 in, 6 out]
        n206 = event-data("Accepted?"=w547) -> ()  [unwired: 1 in, 1 out]
      }
      event Panel Close? {
        # "Intercepts the upper right close panel operation to allow a smooth shutdown as opposed to immediately killing the app."
        n207 = event-data() -> ()  [unwired: 1 in, 1 out]
        n208 = call <vilib>:"Send Local Message.vi"("message queue in"=w556, "message name"="Close?", "error in"=w553) -> ("message queue out"=w554:T4, "error out"=w552:errorcluster)  [unwired: 10 in, 1 out]
        n209 = event-data("Discard?"=TRUE) -> ()  [unwired: 1 in, 1 out]
      }
      event Menu Selection (User) {
        # "#USERCFG It is needed to add a Case for Every item on the menu"
        n210 = event-data() -> ("ItemPath"=w562:string)  [unwired: 1 in]
        n211 = case shown="\"_Tools:Multiple Parameter Editor\"" w562 {
          tunnel: w561 -> [w564 w570 w575 w580 w585 w590 w599]
          tunnel: [w564 w566 w571 w576 w581 w586 w596] -> w560
          tunnel: w559 -> [w563 w568 w573 w578 w583 w588 w595]
          tunnel: [w563 w567 w572 w577 w582 w587 w593] -> w558
          frame Default {
            n212 = One Button Dialog(message="Unknown Menu Option") -> ()  [unwired: 1 in, 1 out]
          }
          frame "_File:_New" {
            n213 = call <vilib>:"Send Local Message.vi"("message queue in"=w570, "message name"="New?" ("Message Name"), "error in"=w568) -> ("message queue out"=w566:T4, "error out"=w567:errorcluster)  [unwired: 10 in, 1 out]
          }
          frame "_File:_Open" {
            n214 = call <vilib>:"Send Local Message.vi"("message queue in"=w575, "message name"="Open?" ("Message Name"), "error in"=w573) -> ("message queue out"=w571:T4, "error out"=w572:errorcluster)  [unwired: 10 in, 1 out]
          }
          frame "_File:_Save" {
            n215 = call <vilib>:"Send Local Message.vi"("message queue in"=w580, "message name"="Save" ("Message Name"), "error in"=w578) -> ("message queue out"=w576:T4, "error out"=w577:errorcluster)  [unwired: 10 in, 1 out]
          }
          frame "_File:Save As..." {
            n216 = call <vilib>:"Send Local Message.vi"("message queue in"=w585, "message name"="SaveAs" ("Message Name"), "error in"=w583) -> ("message queue out"=w581:T4, "error out"=w582:errorcluster)  [unwired: 10 in, 1 out]
          }
          frame "_File:_Exit" {
            n217 = call <vilib>:"Send Local Message.vi"("message queue in"=w590, "message name"="Close?" ("Message Name"), "error in"=w588) -> ("message queue out"=w586:T4, "error out"=w587:errorcluster)  [unwired: 10 in, 1 out]
          }
          frame "_Tools:Multiple Parameter Editor" {
            n218 = call <vilib>:"Send Local Message.vi"("message queue in"=w599, "message name"="CleansubPanel", "error in"=w595) -> ("message queue out"=w598:T4, "error out"=w594:errorcluster)  [unwired: 10 in, 1 out]
            n219 = call <vilib>:"Send Local Message.vi"("message queue in"=w598, "message name"="Custom View" ("Message Name"), "message value"="Multiple Variable Editor" ("Message Name"), "error in"=w594) -> ("message queue out"=w596:T4, "error out"=w593:errorcluster)  [unwired: 9 in, 1 out]
          }
        }
      }
    }
    n220 = call "Error.vi"("error in (no error)"=w388, "message queue in"=w389) -> ()  [unwired: 9 in, 1 out]
  }
